vi "extractBodyOpenCVIP.vi"(3 "minImageNumber":i32) -> (1 "found fly":bool)   [LabVIEW 2012]
uses:
  OpenCvGlobals.vi
  <userlib>/OpenCVImProc/CatWalkLabviewDLLd.dll
  <userlib>/OpenCVImProc/CatWalkLabviewDLL.dll
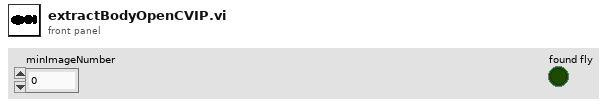
[diagram p1: front panel]
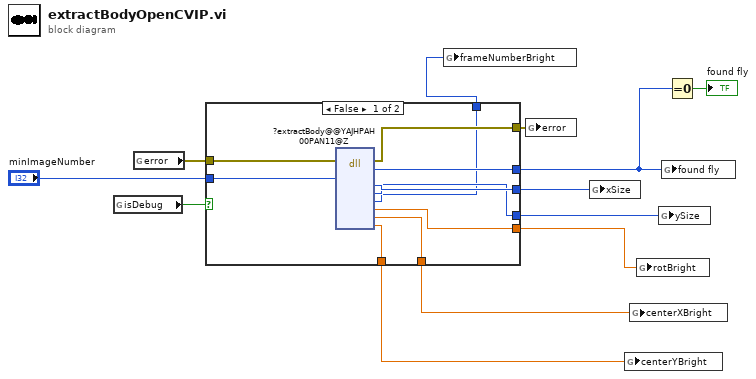
[diagram p0: block diagram]
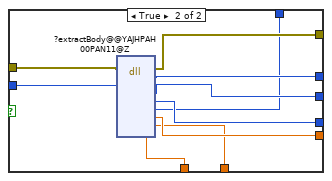
[diagram p2: hidden frame]
diagram:
  n1 = global read "OpenCvGlobals.vi" "isDebug"() -> (w12:bool)
  n2 = global read "OpenCvGlobals.vi" "error"() -> (w10:errorcluster)
  n3 = case shown="False" w12 {
    tunnel: [w21 w30] -> w2
    tunnel: [w18 w31] -> w11
    tunnel: w10 -> [w22 w32]
    tunnel: [w20 w29] -> w9
    tunnel: [w19 w28] -> w8
    tunnel: [w17 w27] -> w7
    tunnel: [w16 w26] -> w6
    tunnel: [w15 w25] -> w5
    tunnel: [w14 w24] -> w4
    tunnel: "minImageNumber" -> [w13 w23]
    frame False {
      n4 = dll-call lib="C:/Program Files (x86)/National Instruments/LabVIEW 2012/user.lib/OpenCVImProc/CatWalkLabviewDLL.dll" fn="?extractBody@@YAJHPAH00PAN11@Z"(error in=w22, "minImageNumber"=w13) -> (error out=w18:errorcluster, "return type"=w21:i32, "xSize"=w20:i32, "ySize"=w19:i32, "frameNumberBright"=w14:i32, "rotBright"=w17:dbl, "centerXBright"=w16:dbl, "centerYBright"=w15:dbl)  [unwired: 9 in, 1 out]
    }
    frame True {
      n5 = dll-call lib="C:/Program Files (x86)/National Instruments/LabVIEW 2012/user.lib/OpenCVImProc/CatWalkLabviewDLLd.dll" fn="?extractBody@@YAJHPAH00PAN11@Z"(error in=w32, "minImageNumber"=w23) -> (error out=w31:errorcluster, "return type"=w30:i32, "xSize"=w29:i32, "ySize"=w28:i32, "frameNumberBright"=w24:i32, "rotBright"=w27:dbl, "centerXBright"=w26:dbl, "centerYBright"=w25:dbl)  [unwired: 9 in, 1 out]
    }
  }
  n6 = global write "OpenCvGlobals.vi" "frameNumberBright"(w4) -> ()
  n7 = global write "OpenCvGlobals.vi" "error"(w11) -> ()
  n8 = global write "OpenCvGlobals.vi" "xSize"(w9) -> ()
  n9 = global write "OpenCvGlobals.vi" "centerYBright"(w5) -> ()
  n10 = global write "OpenCvGlobals.vi" "centerXBright"(w6) -> ()
  n11 = global write "OpenCvGlobals.vi" "rotBright"(w7) -> ()
  n12 = global write "OpenCvGlobals.vi" "ySize"(w8) -> ()
  n13 = global write "OpenCvGlobals.vi" "found fly"(w2) -> ()
  n14 = Equal To 0?(x=w2) -> (x = 0?=→"found fly":bool)
